vi "New Round.vi"(7 "Round":u32, 11 "MyTeam in":refnum<class "MyTeam.lvclass">) -> (3 "MyTeam out":refnum<class "MyTeam.lvclass">)   [LabVIEW 2020, in "Galaxy.lvlib" / "MyTeam.lvclass"]
doc: "This VI is called once at the beginning of each new round. This can be used to do global map updates, coordinated plans for all active squares, or nothing at all!"
uses:
  MyTeam.lvclass
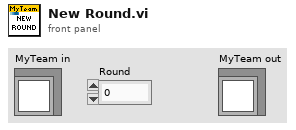
[diagram p1: front panel]
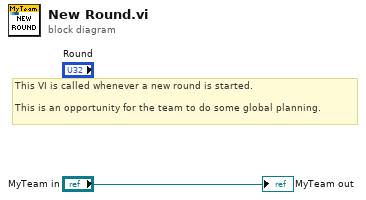
[diagram p0: block diagram]
diagram:
  # "This VI is called whenever a new round is started.\n\nThis is an opportunity for the team to do some global planning."
  "MyTeam out" <- "MyTeam in"
